vi "整合数据9.vi"(0 "Data in":u8[](array[numeric])) -> (2 "P1":i16, 3 "I1":i16, 4 "D1":i16, 6 "P2":i16, 8 "I2":i16, 10 "D2":i16, 13 "D3":i16, 14 "I3":i16, 15 "P3":i16)   [LabVIEW 2016]
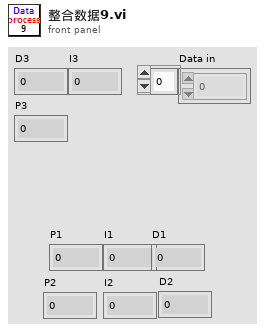
[diagram p1: front panel]
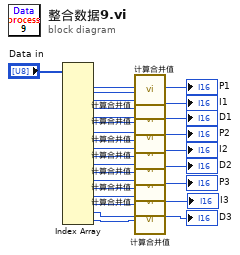
[diagram p0: block diagram]
diagram:
  n1 = Index Array(array="Data in") -> (element #1=w18:u8, element #2=w17:u8, element #3=w16:u8, element #4=w15:u8, element #5=w14:u8, element #6=w13:u8, element #7=w12:u8, element #8=w11:u8, element #9=w10:u8, element #10=w9:u8, element #11=w8:u8, element #12=w7:u8, element #13=w6:u8, element #14=w5:u8, element #15=w4:u8, element #16=w3:u8, element #17=w2:u8, element #18=w1:u8)  [unwired: 18 in]
  n2 = call "计算合并值.vi"("数值H"=w18, "数值L"=w17) -> ("合并数值"=→"P1":i16)  [unwired: 17 in]
  n3 = call "计算合并值.vi"("数值H"=w16, "数值L"=w15) -> ("合并数值"=→"I1":i16)  [unwired: 17 in]
  n4 = call "计算合并值.vi"("数值H"=w14, "数值L"=w13) -> ("合并数值"=→"D1":i16)  [unwired: 17 in]
  n5 = call "计算合并值.vi"("数值H"=w12, "数值L"=w11) -> ("合并数值"=→"P2":i16)  [unwired: 17 in]
  n6 = call "计算合并值.vi"("数值H"=w10, "数值L"=w9) -> ("合并数值"=→"I2":i16)  [unwired: 17 in]
  n7 = call "计算合并值.vi"("数值H"=w8, "数值L"=w7) -> ("合并数值"=→"D2":i16)  [unwired: 17 in]
  n8 = call "计算合并值.vi"("数值H"=w6, "数值L"=w5) -> ("合并数值"=→"P3":i16)  [unwired: 17 in]
  n9 = call "计算合并值.vi"("数值H"=w4, "数值L"=w3) -> ("合并数值"=→"I3":i16)  [unwired: 17 in]
  n10 = call "计算合并值.vi"("数值H"=w2, "数值L"=w1) -> ("合并数值"=→"D3":i16)  [unwired: 17 in]
